vi "Setup For Triggered Images v4.2.vi"(4 "error in":errorcluster caption="error in (no error)", 5 "Timeout (ms)":u32=1000, 6 "Gain":dbl=1000.0, 7 "Shutter Speed (us)":dbl=1000.0, 8 "Camera Name":T3) -> (0 "Error out":errorcluster caption="error in (no error)", 1 "Session Out":T3, 2 "Height":u32, 3 "Width":u32)   [LabVIEW 2013]
doc: "The Grab and Attributes Setup VI acquires images continuously and displays the images in an image control using high-level acquisition VIs. The VI also modifes the camera attributes while acquiring images. A grab is appropriate for high-speed applications in which you need to process only one image at a time."
uses:
  <vilib>/userdefined/High Color/IMAQdx.ctl
  <vilib>/vision/driver/IMAQdx.llb/IMAQdx Attribute Type.ctl
  <vilib>/vision/driver/IMAQdx.llb/IMAQdx Attribute Visibility.ctl
  <vilib>/vision/driver/IMAQdx.llb/IMAQdx Acquisition Mode.ctl
  <vilib>/vision/driver/NI_Vision_Acquisition_Software.lvlib
  <resource>/objmgr/imaqdx.rc
panel:
  out "PixelFormat":u32
  out "Attribute Information Array":T2(array[cluster])
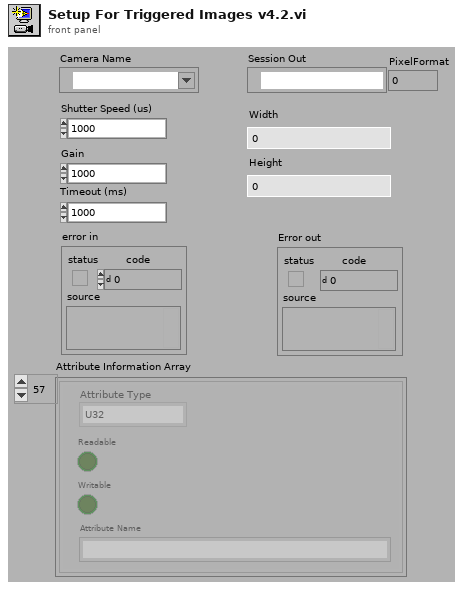
[diagram p1: front panel]
types:
  T1 = typedef "NI_Vision_Acquisition_Software.lvlib/IMAQdx Attribute Type.ctl" = enum32{"U32", "I64", "DBL", "String", "Enum", "Bool", "Command"}
  T2 = cluster{"Attribute Type":T1, "Readable":bool, "Writable":bool, "Attribute Name":string}[]
  T3 = typedef "IMAQdx.ctl" = refnum<k21>
  T4 = typedef "NI_Vision_Acquisition_Software.lvlib/IMAQdx Attribute Visibility.ctl" = enum32{"Simple", "Intermediate", "Advanced"}
  T5 = typedef "NI_Vision_Acquisition_Software.lvlib/IMAQdx Acquisition Mode.ctl" = enum32{"One Shot", "Continuous"}
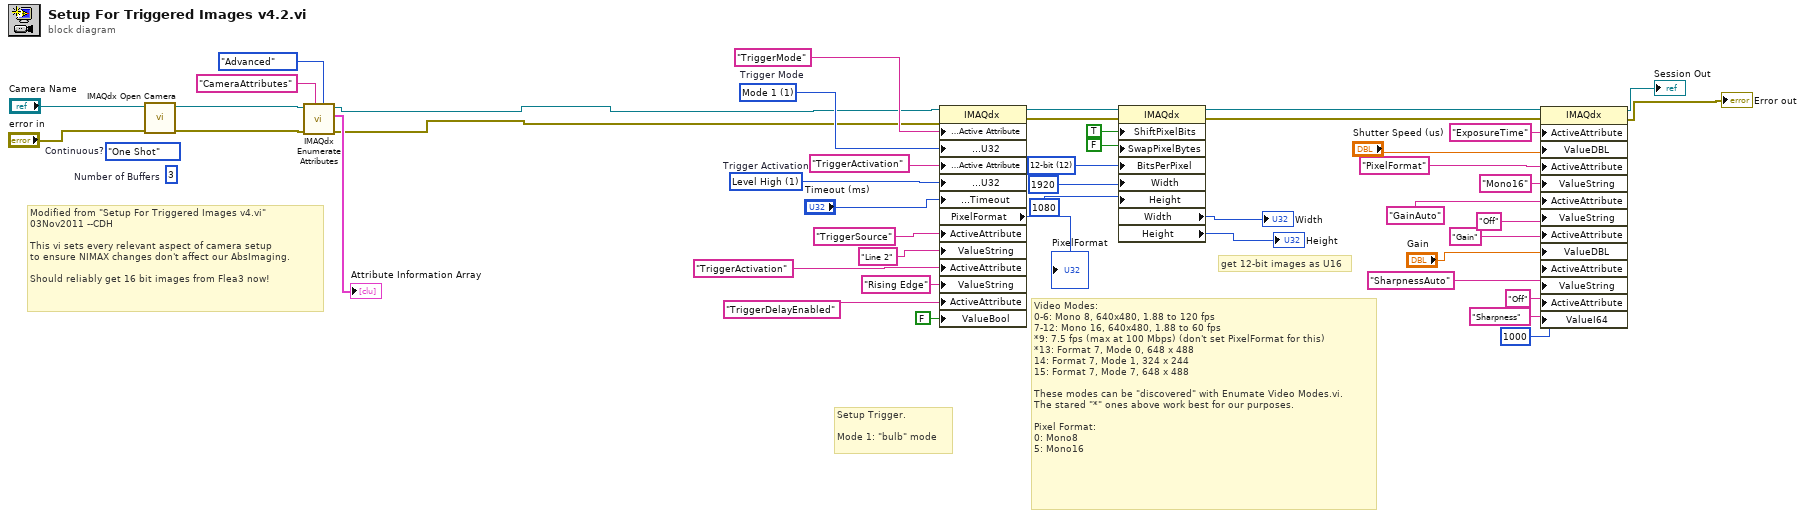
[diagram p0: block diagram]
diagram:
  w32 = u32 12 items=["Use Hardware Value"=0, "10-bit"=10, "12-bit"=12, "14-bit"=14, "16-bit"=16] ("BitsPerPixel")
  w41 = u32 1 items=["Mode 0"=0, "Mode 1"=1, "Mode 3"=3, "Mode 14"=14, "Mode 15"=15, "Off"=16]  # Trigger Mode
  w40 = u32 1 items=["Level Low", "Level High"]  # Trigger Activation
  (unwired) u32 3  # Number of Buffers
  (unwired) IMAQdx_Acquisition_Mode."One Shot"  # Continuous?
  # "Modified from \"Setup For Triggered Images v4.vi\"\n03Nov2011 --CDH\n\nThis vi sets every relevant aspect of camera setup\nto ensure NIMAX changes don't affect our AbsImaging.\n\nShould reliably get 16 bit images from Flea3 now!"
  # "get 12-bit images as U16"
  # "Video Modes:\n0-6: Mono 8, 640x480, 1.88 to 120 fps\n7-12: Mono 16, 640x480, 1.88 to 60 fps\n*9: 7.5 fps (max at 100 Mbps) (don't set PixelFormat for this)\n*13: Format 7, Mode 0, 648 x 488\n14: Format 7, Mode 1, 324 x 244\n15: Format 7, Mode 7, 648 x 488 \n\nThese modes can be \"discovered\" with Enumate Video Modes.vi.\nThe stared \"*\" ones above work best for our purposes.\n\nPixel Format:\n0: Mono8\n5: Mono16"
  # "Setup Trigger.\n\nMode 1: \"bulb\" mode"
  n1 = call <vilib>:"IMAQdx Open Camera.vi"("error in"="error in", "Session In"="Camera Name") -> ("error out"=w34:errorcluster, "Session Out"=w35:T3)  [unwired: 1 in, 7 out]
  n2 = call <vilib>:"IMAQdx Enumerate Attributes.vi"("Visibility"=IMAQdx_Attribute_Visibility."Advanced", "Root"="CameraAttributes", "error in"=w34, "Session In"=w35) -> ("error out"=w3:errorcluster, "Attribute Information Array"=→"Attribute Information Array":T2, "Session Out"=w4:T3)  [unwired: 5 out]
  n3 = property class="IMAQdx"(reference=w4, error in=w3, "Camera Attributes:Active Attribute"="TriggerMode" ("ActiveAttribute"), "Camera Attributes:Value:U32"=w41, "Camera Attributes:Active Attribute"="TriggerActivation" ("ActiveAttribute"), "Camera Attributes:Value:U32"=w40, "Acquisition Attributes:Timeout"="Timeout (ms)", "ActiveAttribute"="TriggerSource", "ValueString"="Line 2", "ActiveAttribute"="TriggerActivation", "ValueString"="Rising Edge", "ActiveAttribute"="TriggerDelayEnabled", "ValueBool"=FALSE) -> (reference out=w38:T3, error out=w37:errorcluster, "PixelFormat"=→"PixelFormat":u32)
  n4 = property class="IMAQdx"(reference=w38, error in=w37, "ShiftPixelBits"=TRUE, "SwapPixelBytes"=FALSE, "BitsPerPixel"=w32, "Width"=u32 1920, "Height"=u32 1080) -> (reference out=w25:T3, error out=w23:errorcluster, "Width"=→"Width":u32, "Height"=→"Height":u32)
  n5 = property class="IMAQdx"(reference=w25, error in=w23, "ActiveAttribute"="ExposureTime", "ValueDBL"="Shutter Speed (us)", "ActiveAttribute"="PixelFormat", "ValueString"="Mono16", "ActiveAttribute"="GainAuto", "ValueString"="Off", "ActiveAttribute"="Gain", "ValueDBL"="Gain", "ActiveAttribute"="SharpnessAuto", "ValueString"="Off", "ActiveAttribute"="Sharpness", "ValueI64"=i64 1000) -> (reference out=→"Session Out":T3, error out=→"Error out":errorcluster)
